vi "AH2500_write_data.vi"(7 "File reference":refnum<file>) -> ()   [LabVIEW 2019]
uses:
  Global/Global Variables/Data_Display_global.vi
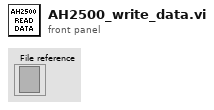
[diagram p1: front panel]
types:
  T1 = typedef "AH2500-Cluster.ctl" = cluster{"Capacity Graphic":dbl[][], "Loss Graphic":dbl[][], "Update AH2500":bool, "Capacity":dbl, "Loss":dbl, "AVerage":enum16{"0", "1", "2", "3", "4", "5", "6", "7", "8", "9", "10", "11", "12", "13", "14", "15"}, "ALternate":enum16{"0", "1", "2", "3", "4", "5", "6", "7"}, "BIas":enum16{"Disabled", "100 MOhm", "1 MOhm"}, "V excitation":enum16{"15.00", "7.50", "3.75", "3.00", "1.50", "0.750", "0.375", "0.250", "0.125", "0.100", "0.050", "0.030", "0.015", "0.010", "0.0050", "0.0030", "0.0015", "0.0010", "0.0005"}}
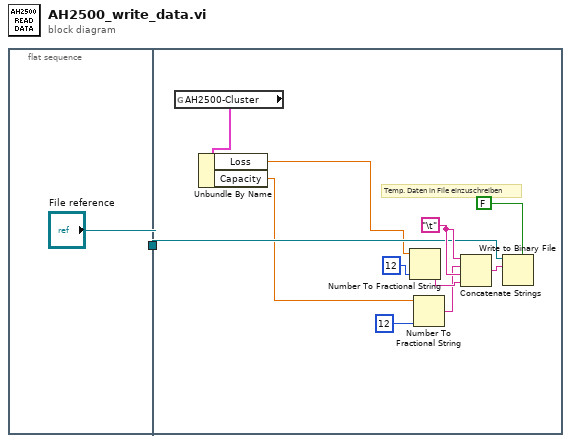
[diagram p0: block diagram]
diagram:
  n1 = flat-sequence {
    tunnel: ["File reference"] -> w1
    tunnel: w1 -> [w6]
    frame #0 {
    }
    frame #1 {
      w11 = "\t"
      # "Temp. Daten in File einzuschreiben"
      n2 = global read "Data_Display_global.vi" "AH2500-Cluster"() -> (w5:T1)
      n3 = Unbundle By Name(w5) -> ("Loss"=w4:dbl, "Capacity"=w3:dbl)
      n4 = Number To Fractional String(number=w4, precision (6)=i16 12) -> (F-format string=w12:string)  [unwired: 2 in]
      n5 = Number To Fractional String(number=w3, precision (6)=i16 12) -> (F-format string=w8:string)  [unwired: 2 in]
      n6 = Concatenate Strings(w11, w8, w11, w12) -> (w13:string)
      n7 = Write to Binary File ("Write File")(file (use dialog)=w6, data=w13, 5:FALSE ("prepend array or string size? (T)")) -> ()  [unwired: 3 in, 3 out]
    }
  }
